vi "HFRR ADV v05.vi"() -> ()   [LabVIEW 2025] (continued)
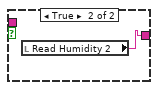
[diagram p4: hidden frame]
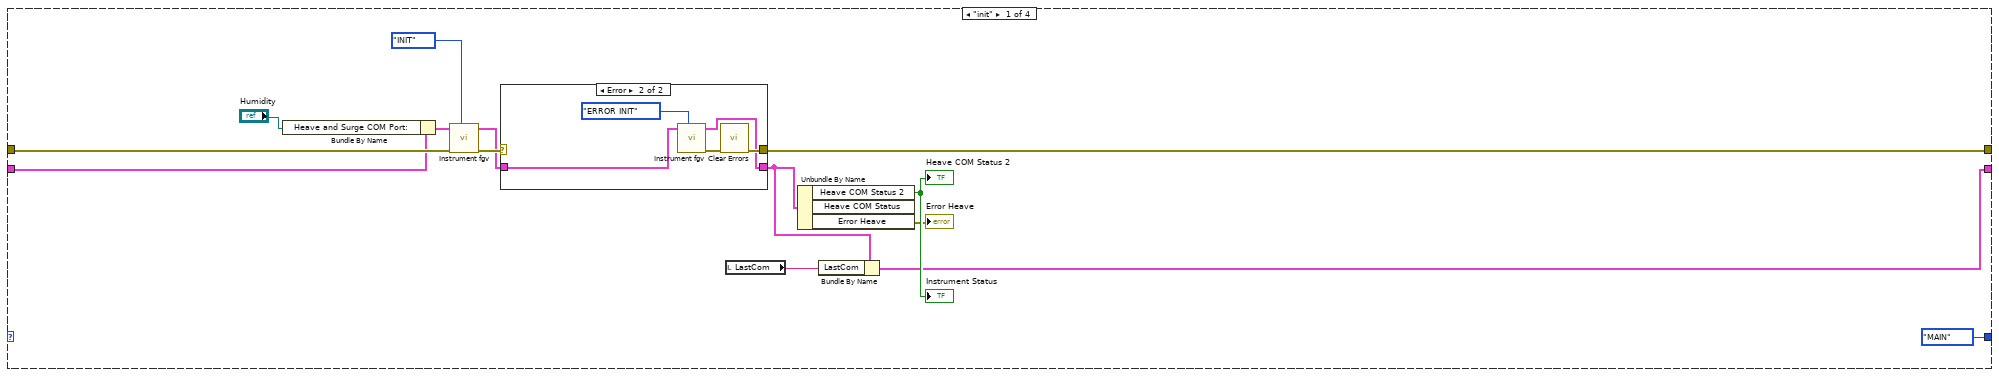
[diagram p5: hidden frame]
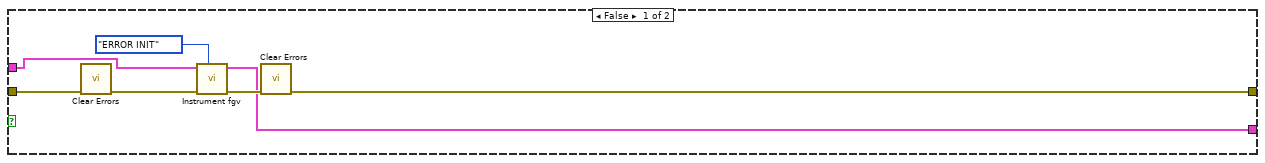
[diagram p7: hidden frame]
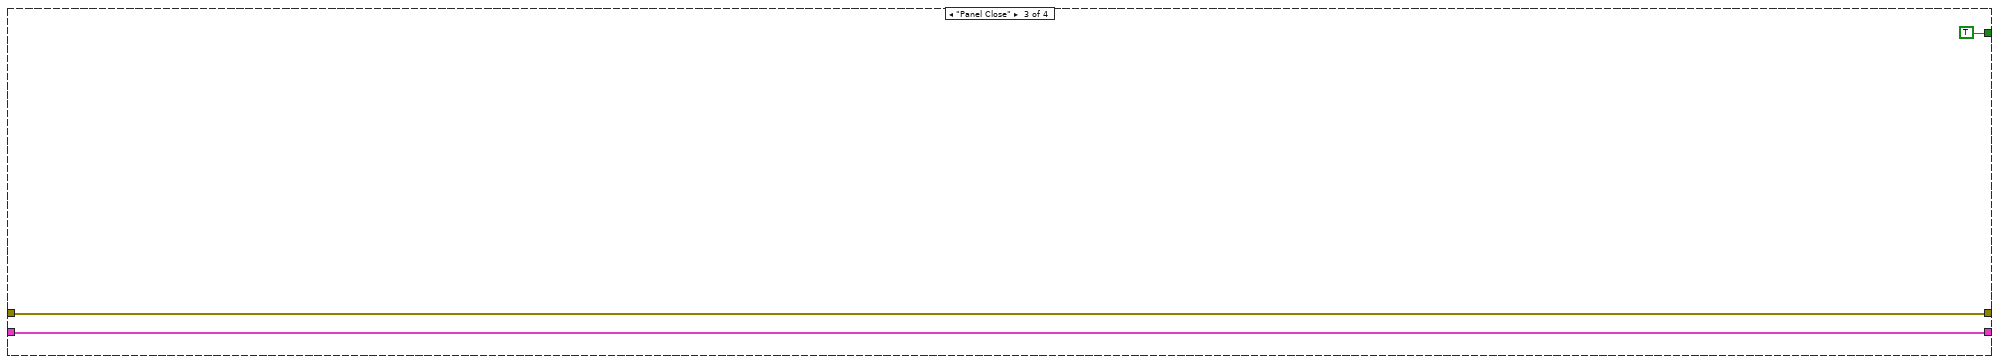
[diagram p11: hidden frame]
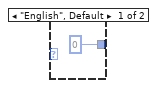
[diagram p13: hidden frame]
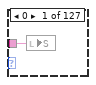
[diagram p14: hidden frame]
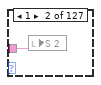
[diagram p15: hidden frame]
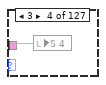
[diagram p17: hidden frame]
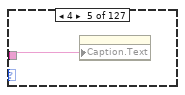
[diagram p18: hidden frame]
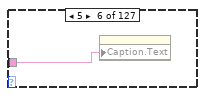
[diagram p19: hidden frame]
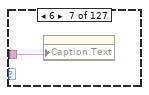
[diagram p20: hidden frame]
          tunnel: [w4833] -> w4737
          frame #0 {
            n3292 = Wait (ms)(milliseconds to wait=u32 50) -> ()  [unwired: 1 out]
          }
        }
        n3293 = case shown="No Error" w4737 {
          selector: w4737 -> [w4783 w4826]
          tunnel: w4741 -> [w4782 w4825]
          tunnel: [w4749 w4816] -> w4740
          tunnel: [w4750 w4824] -> w4739
          frame No Error {
            w4776 = T21 {"Mode"=enum."RTU", "Slave Address"=1} ("Serial Parameters")
            n3294 = call-poly <vilib>:"MB Serial Master Query (poly).vi"("VISA resource name"=w4782, "Starting Address"=i16 1000, "Quantity"=u16 1, "Timeout"=u32 1000, "error in"=w4783, "Serial Parameters"=w4776) -> ("VISA resource name out"=w4777:refnum<visa-resource-name>, "Input Registers"=w4779:u16[], "error out"=w4775:errorcluster)  [unwired: 10 in, 1 out]
            n3295 = Random Number (0-1)() -> (number: 0 to 1=w4764:dbl)
            n3296 = Index Array(array=w4779, index=0) -> (element=w4774:u16)
            n3297 = Subtract(x=w4764, y=0.5) -> (x-y=w4763:dbl)
            n3298 = Divide(x=w4774, y=10 ("index")) -> (x/y=w4768:dbl)
            n3299 = Multiply(x=w4763, y=0.5) -> (x*y=w4762:dbl)
            n3300 = Add(x=w4768, y=w4762) -> (x+y=w4767:dbl)
            n3301 = local read "Amb temp"() -> (w4751:dbl)
            n3302 = Multiply(x=w4767, y=0.2) -> (x*y=w4771:dbl)
            n3303 = Multiply(x=w4751, y=0.8) -> (x*y=w4769:dbl)
            n3304 = Add(x=w4771, y=w4769) -> (x+y=w4752:dbl)
            n3305 = local read "set temp old"() -> (w4746:dbl)
            n3306 = local write "Amb temp"(w4752) -> ()
            n3307 = Select(t="SetTemp 2", s="Heater", f=100.0) -> (s? t:f=w4747:dbl)
            n3308 = Not Equal?(x=w4747, y=w4746) -> (x != y?=w4745:bool)
            n3309 = case shown="True" w4745 {
              tunnel: w4777 -> [w4811 w4813]
              tunnel: [w4810 w4813] -> w4757
              tunnel: w4775 -> [w4809 w4812]
              tunnel: [w4808 w4812] -> w4755
              tunnel: w4747 -> [w4803 _]
              tunnel: w4776 -> [w4805 w4814]
              tunnel: [w4805 w4814] -> w4758
              frame True {
                n3310 = Multiply(x=w4803, y=10 ("index")) -> (x*y=w4802:dbl)
                n3311 = call-poly <vilib>:"MB Serial Master Query (poly).vi"("VISA resource name"=w4811, "Address"=u16 0, "Holding Register"=w4802, "Timeout"=u32 1000, "error in"=w4809, "Serial Parameters"=w4805) -> ("VISA resource name out"=w4810:refnum<visa-resource-name>, "error out"=w4808:errorcluster)  [unwired: 11 in, 1 out]
                "set temp old" <- w4803
              }
              frame False {
              }
            }
            n3312 = flat-sequence {
              tunnel: [w4784] -> _
              tunnel: [w4784] -> w4754
              tunnel: w4755 -> [w4784]
              frame #0 {
                n3313 = Wait (ms)(milliseconds to wait=u32 100) -> ()  [unwired: 1 out]
              }
            }
            n3314 = call "Elapsed Time12"("Time Target (s)"=2.0, "Auto Reset"=TRUE) -> ("Time has Elapsed"=w4759:bool)  [unwired: 10 in, 7 out]
            n3315 = case shown="True" w4759 {
              tunnel: w4758 -> [w4788 w4801]
              tunnel: [w4788 w4801] -> _
              tunnel: [w4787 w4799] -> w4750
              tunnel: w4757 -> [w4787 w4800]
              tunnel: [w4786 w4797] -> w4749
              tunnel: w4754 -> [w4786 w4798]
              frame False {
              }
              frame True {
                n3316 = call-poly <vilib>:"MB Serial Master Query (poly).vi"("VISA resource name"=w4800, "Starting Address"=i16 1003 ("Addr"), "Quantity"=u16 1, "Timeout"=u32 1000, "error in"=w4798, "Serial Parameters"=w4801) -> ("VISA resource name out"=w4799:refnum<visa-resource-name>, "Input Registers"=w4794:u16[], "error out"=w4797:errorcluster)  [unwired: 10 in, 1 out]
                n3317 = Index Array(array=w4794, index=0) -> (element=w4793:u16)
                n3318 = Divide(x=w4793, y=u16 10) -> (x/y=w4789:dbl)
                n3319 = local write "set temp old"(w4789) -> ()
                n3320 = local write "SetTemp"(w4789) -> ()
              }
            }
            "Error Code" <- w4749
            n3321 = Unbundle(w4749) -> ("status"=→"TK4 status":bool)  [unwired: 2 out]
            "SetTemp" <- "SetTemp 2"
          }
          frame Error {
            w4828 = u16 0 items=["None", "Odd", "Even", "Mark", "Space"] ("Parity")
            w4829 = u16 0 items=["None", "XON/XOFF", "RTS/CTS", "XON/XOFF & RTS/CTS", "DTR/DSR", "XON/XOFF & DTR/DSR"] ("Flow Control")
            n3322 = VISA Clear(VISA resource name=w4825, error in (no error)=w4826) -> (VISA resource name out=w4819:refnum<visa-resource-name>, error out=w4817:errorcluster)
            n3323 = VISA Close(VISA resource name=w4819, error in (no error)=w4817) -> (error out=w4818:errorcluster)
            n3324 = call <vilib>:"Clear Errors.vi"("error in (no error)"=w4818) -> ("error out"=w4827:errorcluster)  [unwired: 5 in, 1 out]
            n3325 = Unbundle By Name(T21 {"Mode"=enum."RTU", "Slave Address"=1} ("input cluster")) -> ("Mode"=w4830:enum16{"RTU", "ASCII"})
            n3326 = call <vilib>:"MB Serial Init.vi"("Timeout"=u32 100, "Flow Control"=w4829, "Mode"=w4830, "error in (no error)"=w4827, "Parity"=w4828, "Baud Rate"=u32 9600, "VISA resource name"="Lubrication System COM Port :") -> ("error out"=w4816:errorcluster, "VISA resource name out"=w4824:refnum<visa-resource-name>)  [unwired: 3 in]
            n3327 = local write "set temp old"(0.0 ("set temp old")) -> ()
            n3328 = Unbundle(w4816) -> ("status"=w4815:bool)  [unwired: 2 out]
            n3329 = case shown="True" w4815 {
              selector: w4815 -> [_ w4832]
              frame False {
              }
              frame True {
                n3330 = local write "TK4 status"(w4832) -> ()
              }
            }
          }
        }
        n3331 = local read "Quit"() -> (w4736:bool)
      }
      n3332 = VISA Close(VISA resource name=w4732, error in (no error)=w4733) -> (error out=w4731:errorcluster)
      n3333 = call <vilib>:"Clear Errors.vi"("error in (no error)"=w4731) -> ()  [unwired: 5 in, 2 out]
    }
    frame Enabled {
    }
  }
  "file count" <- 0 ("file count")
